vi "A Simple Control Panel Example.vi"() -> ()   [LabVIEW 2011]
panel:
  in  "send":bool
  out "Return":string
  in  "Comand":string
  in  "Axis #":u16(ring) items=["1", "2", "3", "4", "5", "6"]
  in  "Zero":bool
  in  "Decel":dbl=0.001 min=0.001 step=0.1 format="%.3f"
  in  "Accel":dbl=0.001 min=0.001 step=0.1 format="%.3f"
  in  "Vel":dbl=0.0001 min=0.0001 step=0.01 format="%.4f"
  in  ">":bool
  in  "<":bool
  in  "increment":dbl=0.5 step=0.001 format="%.6f"
  in  "stop":bool
  in  "Go 2":bool
  in  "Go 1":bool
  in  "target Pos 2":dbl step=0.05 format="%.6f"
  in  "target Pos 1":dbl=2.0 step=0.05 format="%.6f"
  in  "exit":bool
  out "Encoder":dbl format="%.6f"
  out "Position":dbl format="%.6f"
  # "MMC-100"
  # "Simple Control Panel"
  # "Motion"
  # "mm"
  # "mm"
  # "Calc"
  # "mm"
  # "mm"
  # "Enc"
  # "mm"
  # "Terminal"
  # "Motion parameters"
  # "mm/s"
  # "mm/s²"
  # "mm/s²"
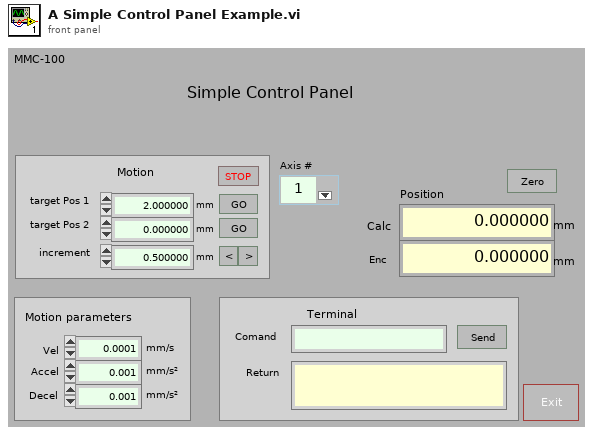
[diagram p1: front panel]
types:
  T1 = cluster{"P type":u16, "VISA resource name out":refnum<visa-resource-name>, " Terminator":string, "Timeout":i32}
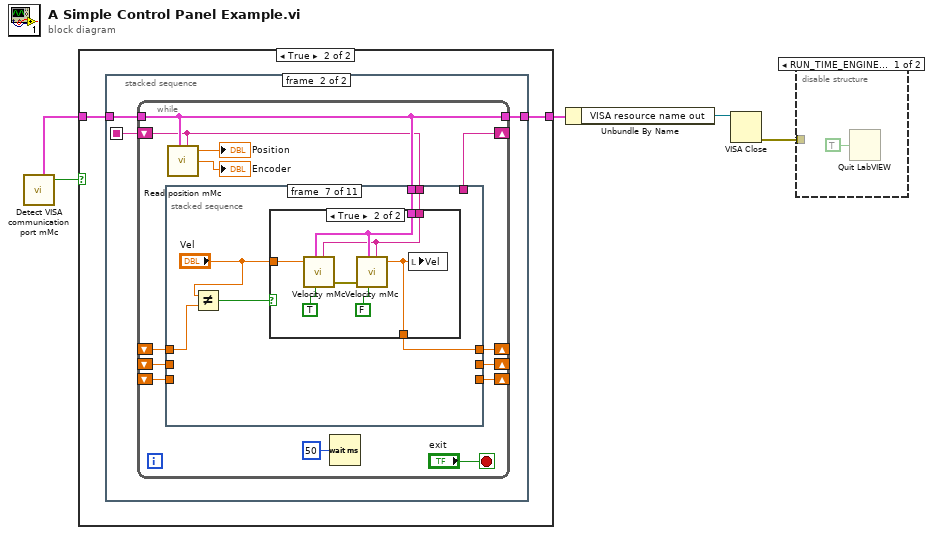
[diagram p0: block diagram]
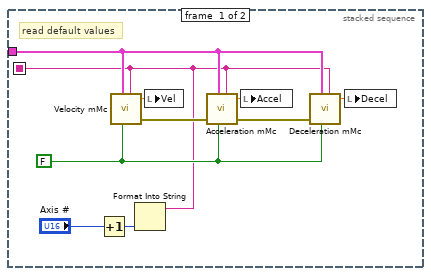
[diagram p4: hidden frame]
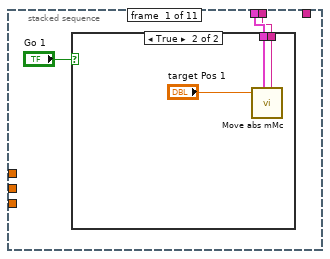
[diagram p5: hidden frame]
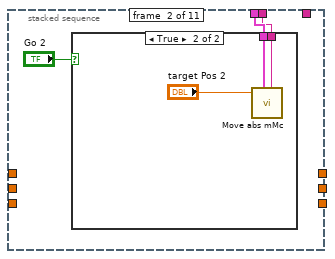
[diagram p7: hidden frame]
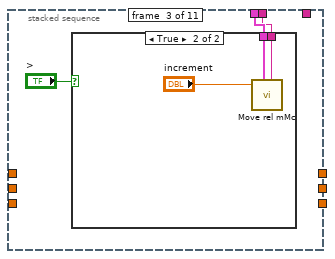
[diagram p9: hidden frame]
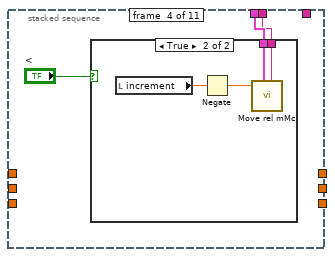
[diagram p11: hidden frame]
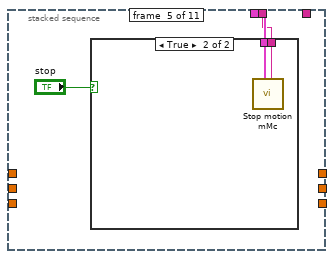
[diagram p13: hidden frame]
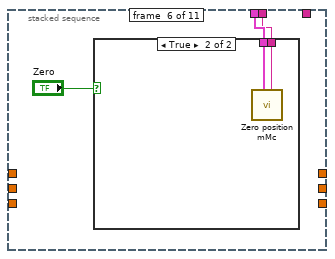
[diagram p15: hidden frame]
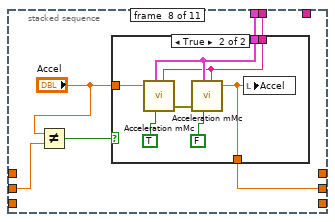
[diagram p18: hidden frame]
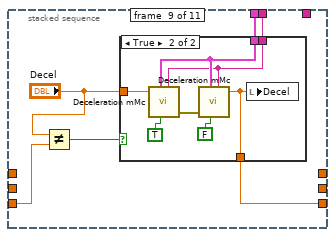
[diagram p20: hidden frame]
diagram:
  n1 = call "Detect VISA communication port mMc.vi"() -> ("Port"=w3:T1, "Port OK"=w4:bool)  [unwired: 6 in, 2 out]
  n2 = case shown="True" w4 {
    tunnel: w3 -> [w6 w8]
    tunnel: [w6 w7] -> w2
    frame False {
    }
    frame True {
      n3 = stacked-sequence {
        seq-local: [w10 _] -> [_ w19]
        tunnel: w8 -> [w15 w21]
        tunnel: [_ w20] -> w7
        frame #0 {
          w18 = FALSE ("set/get")
          # "read default values"
          n4 = Increment(x="Axis #") -> (x+1=w11:u16)
          n5 = Format Into String(w11) -> (resulting string=w10:string)  [unwired: 3 in, 1 out]
          n6 = call "Velocity mMc.vi"("Port"=w15, "set/get"=w18, "Controller #"=w10) -> ("velocity out"=w14:dbl, "error out"=w17:errorcluster)  [unwired: 5 in]
          n7 = local write "Vel"(w14) -> ()
          n8 = call "Acceleration mMc.vi"("Port"=w15, "error in (no error)"=w17, "set/get"=w18, "Controller #"=w10) -> ("accel out"=w13:dbl, "error out"=w16:errorcluster)  [unwired: 4 in]
          n9 = local write "Accel"(w13) -> ()
          n10 = call "Deceleration mMc.vi"("Port"=w15, "error in (no error)"=w16, "set/get"=w18, "Controller #"=w10) -> ("deceleration out"=w12:dbl)  [unwired: 4 in, 1 out]
          n11 = local write "Decel"(w12) -> ()
        }
        frame #1 {
          n12 = while {
            tunnel: w21 -> [w31]
            tunnel: [w31] -> w20
            shift-right: [w29] -> _
            shift-left: _ -> [w30]
            shift-right: [w27] -> _
            shift-left: _ -> [w28]
            shift-right: [w25] -> _
            shift-left: _ -> [w26]
            shift-right: [w22] -> _
            shift-left: w19 -> [w23]
            stop <- "exit" stop-if-true
            n13 = stacked-sequence {
              tunnel: w31 -> [w36 w43 w48 w55 w61 w66 w73 w88 w103 w113 w128]
              tunnel: w23 -> [w35 w42 w47 w54 w60 w65 w72 w89 w102 w116 _]
              tunnel: w30 -> [_ _ _ _ _ _ w75 _ _ _ _]
              tunnel: [_ _ _ _ _ _ w70 _ _ _ _] -> w29
              tunnel: w28 -> [_ _ _ _ _ _ _ w87 _ _ _]
              tunnel: [_ _ _ _ _ _ _ w84 _ _ _] -> w27
              tunnel: w26 -> [_ _ _ _ _ _ _ _ w101 _ _]
              tunnel: [_ _ _ _ _ _ _ _ w98 _ _] -> w25
              tunnel: [_ _ _ _ _ _ _ _ _ w117 _] -> w22
              frame #0 {
                n14 = case shown="True" "Go 1" {
                  tunnel: w36 -> [_ w40]
                  tunnel: w35 -> [_ w39]
                  frame False {
                  }
                  frame True {
                    n15 = call "Move abs mMc.vi"("target pos in"="target Pos 1", "Port"=w40, "Controller #"=w39) -> ()  [unwired: 6 in, 1 out]
                  }
                }
              }
              frame #1 {
                n16 = case shown="True" "Go 2" {
                  tunnel: w43 -> [_ w46]
                  tunnel: w42 -> [_ w45]
                  frame False {
                  }
                  frame True {
                    n17 = call "Move abs mMc.vi"("target pos in"="target Pos 2", "Port"=w46, "Controller #"=w45) -> ()  [unwired: 6 in, 1 out]
                  }
                }
              }
              frame #2 {
                n18 = case shown="True" ">" {
                  tunnel: w48 -> [_ w52]
                  tunnel: w47 -> [_ w51]
                  frame False {
                  }
                  frame True {
                    n19 = call "Move rel mMc.vi"("position incr"="increment", "Port"=w52, "Controller #"=w51) -> ()  [unwired: 6 in, 1 out]
                  }
                }
              }
              frame #3 {
                n20 = case shown="True" "<" {
                  tunnel: w55 -> [_ w59]
                  tunnel: w54 -> [_ w58]
                  frame False {
                  }
                  frame True {
                    n21 = local read "increment"() -> (w57:dbl)
                    n22 = Negate(x=w57) -> (-x=w56:dbl)
                    n23 = call "Move rel mMc.vi"("position incr"=w56, "Port"=w59, "Controller #"=w58) -> ()  [unwired: 6 in, 1 out]
                  }
                }
              }
              frame #4 {
                n24 = case shown="True" "stop" {
                  tunnel: w61 -> [_ w64]
                  tunnel: w60 -> [_ w63]
                  frame False {
                  }
                  frame True {
                    n25 = call "Stop motion mMc.vi"("Port"=w64, "Controller #"=w63) -> ()  [unwired: 7 in, 1 out]
                  }
                }
              }
              frame #5 {
                n26 = case shown="True" "Zero" {
                  tunnel: w66 -> [_ w69]
                  tunnel: w65 -> [_ w68]
                  frame False {
                  }
                  frame True {
                    n27 = call "Zero position mMc.vi"("Port"=w69, "Controller #"=w68) -> ()  [unwired: 7 in, 1 out]
                  }
                }
              }
              frame #6 {
                n28 = Not Equal?(x="Vel", y=w75) -> (x != y?=w74:bool)
                n29 = case shown="True" w74 {
                  tunnel: w73 -> [_ w78]
                  tunnel: w72 -> [_ w77]
                  tunnel: "Vel" -> [w76 w83]
                  tunnel: [w76 w80] -> w70
                  frame False {
                  }
                  frame True {
                    n30 = call "Velocity mMc.vi"("velocity in"=w83, "Port"=w78, "set/get"=TRUE, "Controller #"=w77) -> ("error out"=w81:errorcluster)  [unwired: 4 in, 1 out]
                    n31 = call "Velocity mMc.vi"("Port"=w78, "error in (no error)"=w81, "set/get"=FALSE, "Controller #"=w77) -> ("velocity out"=w80:dbl)  [unwired: 4 in, 1 out]
                    n32 = local write "Vel"(w80) -> ()
                  }
                }
              }
              frame #7 {
                n33 = Not Equal?(x="Accel", y=w87) -> (x != y?=w86:bool)
                n34 = case shown="True" w86 {
                  tunnel: w89 -> [_ w93]
                  tunnel: w88 -> [_ w94]
                  tunnel: "Accel" -> [w90 w97]
                  tunnel: [w90 w91] -> w84
                  frame False {
                  }
                  frame True {
                    n35 = call "Acceleration mMc.vi"("accel in"=w97, "Port"=w94, "set/get"=TRUE, "Controller #"=w93) -> ("error out"=w95:errorcluster)  [unwired: 4 in, 1 out]
                    n36 = call "Acceleration mMc.vi"("Port"=w94, "error in (no error)"=w95, "set/get"=FALSE, "Controller #"=w93) -> ("accel out"=w91:dbl)  [unwired: 4 in, 1 out]
                    n37 = local write "Accel"(w91) -> ()
                  }
                }
              }
              frame #8 {
                n38 = Not Equal?(x="Decel", y=w101) -> (x != y?=w100:bool)
                n39 = case shown="True" w100 {
                  tunnel: w103 -> [_ w106]
                  tunnel: w102 -> [_ w105]
                  tunnel: "Decel" -> [w104 w111]
                  tunnel: [w104 w107] -> w98
                  frame False {
                  }
                  frame True {
                    n40 = call "Deceleration mMc.vi"("deceleration in"=w111, "Port"=w106, "set/get"=TRUE, "Controller #"=w105) -> ("error out"=w108:errorcluster)  [unwired: 4 in, 1 out]
                    n41 = call "Deceleration mMc.vi"("Port"=w106, "error in (no error)"=w108, "set/get"=FALSE, "Controller #"=w105) -> ("deceleration out"=w107:dbl)  [unwired: 4 in, 1 out]
                    n42 = local write "Decel"(w107) -> ()
                  }
                }
              }
              frame #9 {
                n43 = local read "Axis #"() -> (w112:u16)
                n44 = Increment(x=w112) -> (x+1=w118:u16)
                n45 = Format Into String(w118) -> (resulting string=w114:string)  [unwired: 3 in, 1 out]
                n46 = Not Equal?(x=w114, y=w116) -> (x != y?=w115:bool)
                n47 = case shown="True" w115 {
                  tunnel: [w119 w120] -> w117
                  tunnel: w116 -> [w119 _]
                  tunnel: w114 -> [_ w120]
                  tunnel: w113 -> [_ w121]
                  frame False {
                  }
                  frame True {
                    w122 = FALSE ("set/get")
                    n48 = call "Velocity mMc.vi"("Port"=w121, "set/get"=w122, "Controller #"=w120) -> ("velocity out"=w127:dbl, "error out"=w124:errorcluster)  [unwired: 5 in]
                    n49 = local write "Vel"(w127) -> ()
                    n50 = call "Acceleration mMc.vi"("Port"=w121, "error in (no error)"=w124, "set/get"=w122, "Controller #"=w120) -> ("accel out"=w126:dbl, "error out"=w123:errorcluster)  [unwired: 4 in]
                    n51 = local write "Accel"(w126) -> ()
                    n52 = call "Deceleration mMc.vi"("Port"=w121, "error in (no error)"=w123, "set/get"=w122, "Controller #"=w120) -> ("deceleration out"=w125:dbl)  [unwired: 4 in, 1 out]
                    n53 = local write "Decel"(w125) -> ()
                  }
                }
              }
              frame #10 {
                n54 = case shown="True" "send" {
                  tunnel: w128 -> [_ w130]
                  frame False {
                  }
                  frame True {
                    n55 = call "Communication VISA mMc.vi"("Port"=w130, "Command"="Comand") -> ("Return"=→"Return":string)  [unwired: 4 in, 3 out]
                  }
                }
              }
            }
            n56 = call "Read position mMc.vi"("Port"=w31, "Controller #"=w23) -> ("Cnt pos"=→"Position":dbl, "Enc pos"=→"Encoder":dbl)  [unwired: 5 in, 1 out]
            n57 = Wait (ms)(milliseconds to wait=u32 50) -> ()  [unwired: 1 out]
          }
        }
      }
    }
  }
  n58 = Unbundle By Name(w2) -> ("VISA resource name out"=w5:refnum<visa-resource-name>)
  n59 = VISA Close(VISA resource name=w5) -> (error out=w1:errorcluster)  [unwired: 1 in]
  n60 = disable-structure shown="RUN_TIME_ENGINE==True" {
    disable-tunnel: w1 -> [_ _]
    frame condition #0 {
      n61 = Quit LabVIEW(quit? (T)=TRUE ("stop? (T)")) -> ()
    }
    frame condition #1 (active) {
    }
  }
